vi "Write Class Ref.vi"(10 "Class Ref":refnum<vi>, 11 "Opaque Struct Writer in":refnum<class "Opaque Struct Writer.lvclass">) -> (3 "Opaque Struct Writer out":refnum<class "Opaque Struct Writer.lvclass">)   [LabVIEW 2013, in "Opaque Struct Writer.lvclass"]
uses:
  Opaque Struct Writer.lvclass
  Opaque Struct Writer.lvclass/Opaque Struct Writer.ctl
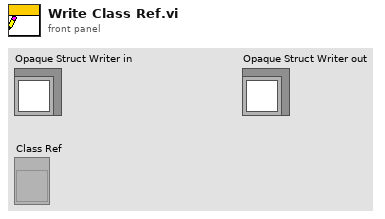
[diagram p1: front panel]
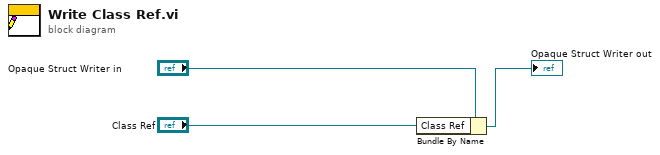
[diagram p0: block diagram]
diagram:
  n1 = Bundle By Name(cluster="Opaque Struct Writer in", "Class Ref"="Class Ref") -> (→"Opaque Struct Writer out":refnum<class "Opaque Struct Writer.lvclass">)
